vi "Reserve(Board).vi"(8 "error in":errorcluster, 11 "ServerRElement":u32) -> (0 "error out":errorcluster, 1 "PortHandles":u32[](array[numeric]), 2 "BoardHandle":u32, 3 "Resources":T1(array[cluster]), 4 "elements found":i32, 5 "found":bool)   [LabVIEW 2020, in "AIM664LV.lvlib"]
doc: "Reserve the specific resource in the end system.s"
uses:
  AIM664LV.lvlib
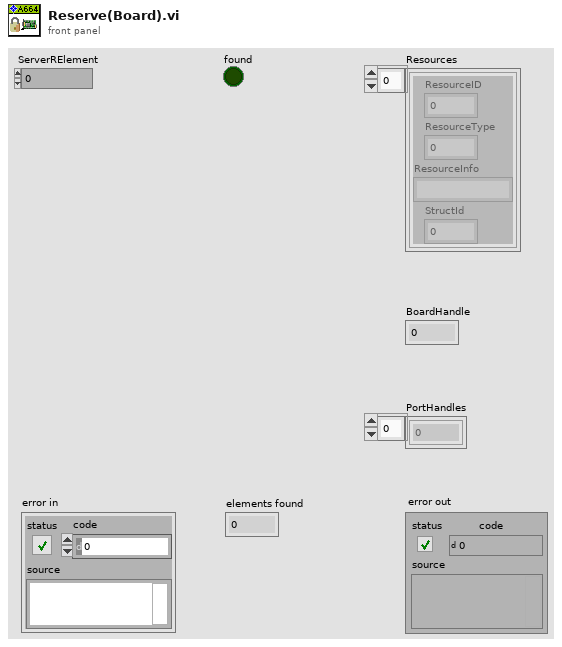
[diagram p1: front panel]
types:
  T1 = cluster{"ResourceID":u32, "ResourceType":u32, "ResourceInfo":string, "StructId":u32}[]
  T2 = cluster{"ResourceID":u32, "ResourceType":u32, "ResourceInfo":string, "StructId":u32}
  T3 = cluster{"BoardName":string, "BoardSerialNo":u32, "BoardNumOf\nEthernetPorts":u32, "BoardClients":u32, "BoardGlobal\nMemSize":u32, "BoardShared\nMemSize":u32, "BoardStructId":u32, "PortName":string, "PortMode":u32, "PortNo":u32, "PortBoard\nResourceID":u32, "PortStructId":u32}
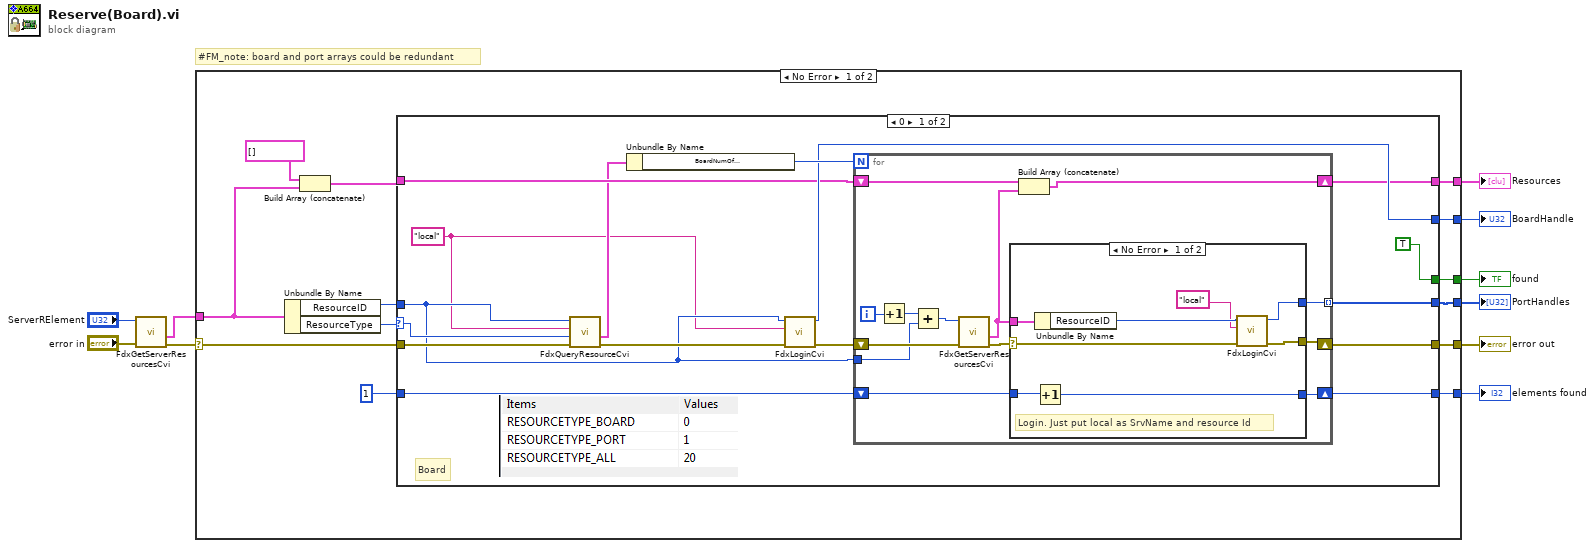
[diagram p0: block diagram]
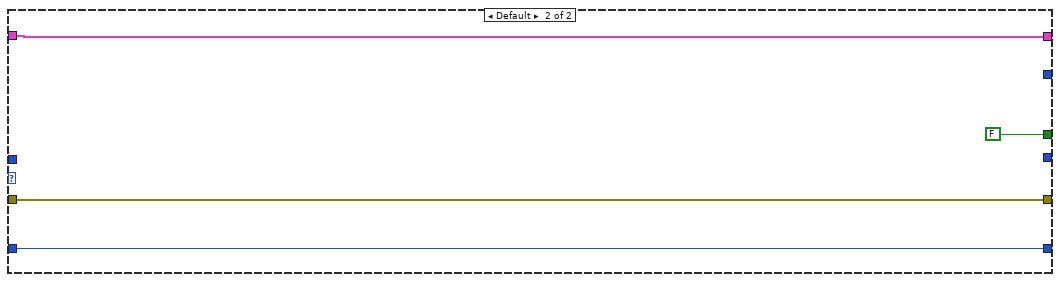
[diagram p3: hidden frame]
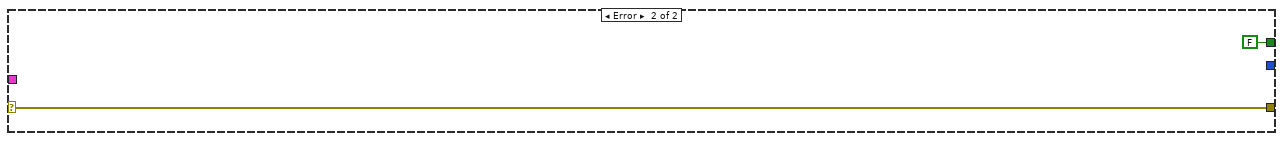
[diagram p4: hidden frame]
diagram:
  # "#FM_note: board and port arrays could be redundant"
  n1 = call "FdxGetServerResourcesCvi.vi"("error in"="error in", "ServerRElement"="ServerRElement") -> ("error out"=w1:errorcluster, "ServerResourceInfo"=w10:T2)  [unwired: 4 in, 4 out]
  n2 = case shown="No Error" w1 {
    selector: w1 -> [w11 w67]
    tunnel: w10 -> [w21 _]
    tunnel: [w19 w67] -> w9
    tunnel: [w17 _] -> w7
    tunnel: [w16 _] -> w6
    tunnel: [w15 _] -> w5
    tunnel: [w14 _] -> w4
    tunnel: [w12 FALSE] -> w2
    frame No Error {
      n3 = Unbundle By Name(w21) -> ("ResourceID"=w22:u32, "ResourceType"=w23:u32)
      n4 = Build Array (concatenate)(T1 [] ("array"), w21) -> (w20:T1)
      n5 = case shown="0" w23 {
        selector: w23 -> [w26 _]
        tunnel: w11 -> [w39 w65]
        tunnel: 1 -> [w32 w66]
        tunnel: w22 -> [w25 _]
        tunnel: [w35 _] -> w16
        tunnel: [w34 w65] -> w19
        tunnel: [w33 _] -> w15
        tunnel: [w31 w66] -> w17
        tunnel: [TRUE FALSE] -> w12
        tunnel: w20 -> [w29 w63]
        tunnel: [w27 w63] -> w14
        frame 0 {
          w24 = "local" ("SrvName")
          # "Board"
          n6 = call "FdxQueryResourceCvi.vi"("error in"=w39, "ResourceType"=w26, "SrvName"=w24, "ResourceID"=w25) -> ("error out"=w37:errorcluster, "ResourceInfo"=w28:T3)  [unwired: 5 in, 1 out]
          n7 = Unbundle By Name(w28) -> ("BoardNumOf\nEthernetPorts"=w38:u32)
          n8 = call "FdxLoginCvi.vi"("error in"=w37, "SrvName"=w24, "ResourceID"=w25) -> ("error out"=w36:errorcluster, "InstrumentHandle"=w33:u32)  [unwired: 7 in]
          n9 = for {
            N: w38 -> [_]
            tunnel: w25 -> [w49]
            shift-right: [w46] -> w34
            shift-left: w36 -> [w52]
            tunnel: [w45] -> w35 mode=indexing
            shift-right: [w43] -> w31
            shift-left: w32 -> [w44]
            shift-right: [w40] -> w27
            shift-left: w29 -> [w42]
            i -> [w51]
            n10 = Increment(x=w51) -> (x+1=w50:i32)
            n11 = Add(x=w50, y=w49) -> (x+y=w48:u32)
            n12 = call "FdxGetServerResourcesCvi.vi"("error in"=w52, "ServerRElement"=w48) -> ("error out"=w47:errorcluster, "ServerResourceInfo"=w41:T2)  [unwired: 4 in, 4 out]
            n13 = case shown="No Error" w47 {
              selector: w47 -> [w60 w62]
              tunnel: [w59 w62] -> w46
              tunnel: [w58 _] -> w45
              tunnel: w41 -> [w57 _]
              tunnel: w44 -> [w56 w61]
              tunnel: [w55 w61] -> w43
              frame No Error {
                # "Login. Just put local as SrvName and resource Id"
                n14 = Unbundle By Name(w57) -> ("ResourceID"=w54:u32)
                n15 = Increment(x=w56) -> (x+1=w55:i32)
                n16 = call "FdxLoginCvi.vi"("error in"=w60, "SrvName"="local", "ResourceID"=w54) -> ("error out"=w59:errorcluster, "InstrumentHandle"=w58:u32)  [unwired: 7 in]
              }
              frame Error {
              }
            }
            n17 = Build Array (concatenate)(w42, w41) -> (w40:T1)
          }
        }
        frame Default {
        }
      }
    }
    frame Error {
    }
  }
  "error out" <- w9
  "Resources" <- w4
  "BoardHandle" <- w5
  "PortHandles" <- w6
  "elements found" <- w7
  "found" <- w2
